vi "relative access path.vi"(11 "Oauth2 in":refnum<class "Oauth2.lvclass">) -> (1 "Token Access Path":string, 2 "Authorization Path":string)   [LabVIEW 2013, in "Oauth2.lvclass"]
uses:
  Oauth2.lvclass
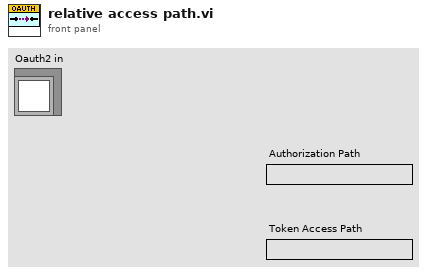
[diagram p1: front panel]
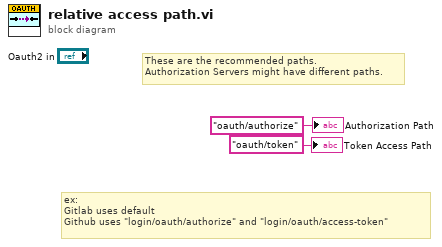
[diagram p0: block diagram]
diagram:
  # "ex: \nGitlab uses default\nGithub uses \"login/oauth/authorize\" and \"login/oauth/access-token\""
  # "These are the recommended paths.\nAuthorization Servers might have different paths."
  "Authorization Path" <- "oauth/authorize" ("Authorization Path")
  "Token Access Path" <- "oauth/token" ("Authorization Path")
